vi "ELVIS III v1.0 Configure AI Mode.vi"(8 "error in (no error)":errorcluster, 10 "AI Channel List":T1, 11 "myRIO FPGA Ref Out":T3) -> (0 "error out":errorcluster)   [LabVIEW 2021]
uses:
  <vilib>/myRIO/Common/Instrument Driver Framework/Utilities/typedefs/Generic FPGA Reference.ctl
  <vilib>/myRIO/Common/Instrument Driver Framework/myRIO v1.0/AI/typedefs/AI Channels List.ctl
  <vilib>/myRIO/Common/Instrument Driver Framework/myRIO v1.0/AI/typedefs/AI Channels Enum.ctl
  <vilib>/myRIO/Common/Instrument Driver Framework/ELVIS III v1.0/AI/typedefs/ELVIS III AI Channels FPGA Reference.ctl
  <vilib>/myRIO/Common/Instrument Driver Framework/ELVIS III v1.0/AI/vis/ELVIS III v1.0 AI Global.vi
  <vilib>/Utility/error.llb/Error Cluster From Error Code.vi
  <vilib>/rvi/errors/niLvFpgaAdjustHostInterfaceError.vi
  <vilib>/rvi/interface/nirviReadWriteControl/nirviReadWriteControl.xnode
  NiFpgaLv.dll
  <vilib>/rvi/interface/Simulation/niFpgaSimulationCallBeginRW.vi
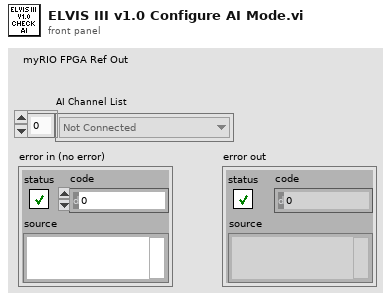
[diagram p1: front panel]
types:
  T1 = typedef "AI Channels List.ctl" = T2[]
  T2 = typedef "AI Channels Enum.ctl" = enum16{"Not Connected", "AudioIn/Left", "AudioIn/Right", "C/AI0", "C/AI1", "A/AI0", "A/AI1", "A/AI2", "A/AI3", "A/AI4", "A/AI5", "A/AI6", "A/AI7", "B/AI0", "B/AI1", "B/AI2", "B/AI3", "B/AI4", "B/AI5", "B/AI6", "B/AI7", "AI/AI0", "AI/AI1", "AI/AI2", "AI/AI3", "A/AI0 (DIFF)", "A/AI1 (DIFF)", "A/AI2 (DIFF)", "A/AI3 (DIFF)", "B/AI0 (DIFF)", "B/AI1 (DIFF)", "B/AI2 (DIFF)", "B/AI3 (DIFF)"}
  T3 = typedef "Generic FPGA Reference.ctl" = refnum<k20>
  T4 = typedef "ELVIS III AI Channels FPGA Reference.ctl" = refnum<k20>
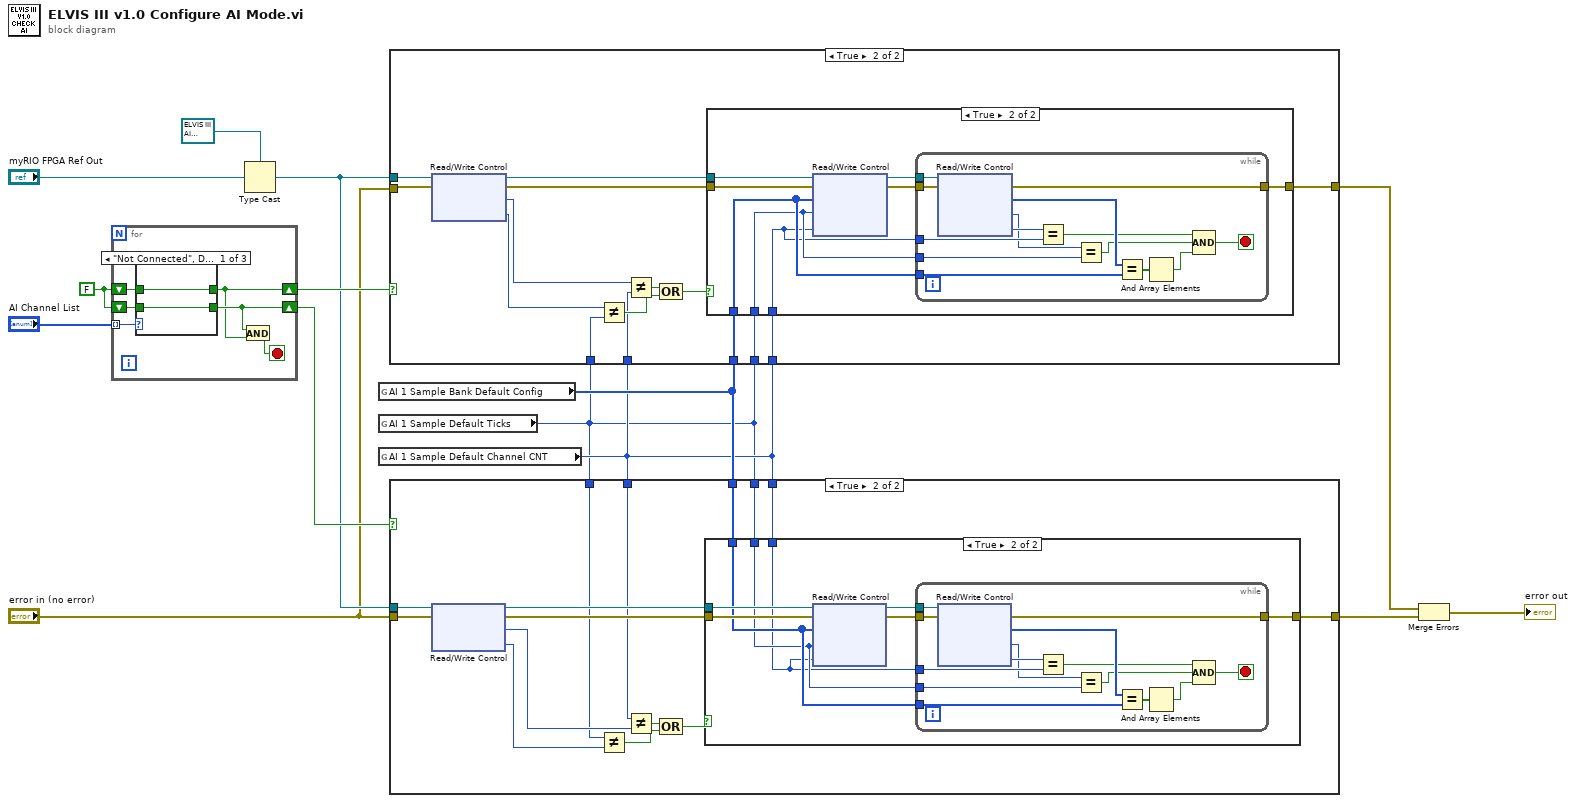
[diagram p0: block diagram]
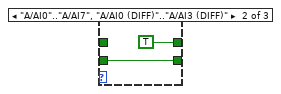
[diagram p6: hidden frame]
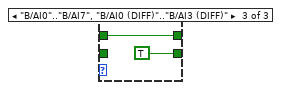
[diagram p7: hidden frame]
diagram:
  w11 = FALSE
  n1 = for {
    tunnel: "AI Channel List" -> [w20] mode=indexing
    shift-right: [w16] -> w10
    shift-left: w11 -> [w18]
    shift-right: [w17] -> w9
    shift-left: w11 -> [w19]
    stop <- w15 stop-if-true
    n2 = case shown="\"Not Connected\", Default" w20 {
      tunnel: w19 -> [w21 w24 _]
      tunnel: [w21 w24 TRUE] -> w17
      tunnel: w18 -> [w22 _ w25]
      tunnel: [w22 TRUE w25] -> w16
      frame "Not Connected", Default {
      }
      frame "A/AI0".."A/AI7", "A/AI0 (DIFF)".."A/AI3 (DIFF)" {
      }
      frame "B/AI0".."B/AI7", "B/AI0 (DIFF)".."B/AI3 (DIFF)" {
      }
    }
    n3 = And(x=w17, y=w16) -> (x .and. y?=w15:bool)
  }
  n4 = Type Cast(type=T4 refnum ("ELVIS III AI Channels FPGA Interface"), x="myRIO FPGA Ref Out") -> (*(type *) &x=w8:T4)
  n5 = global read "ELVIS III v1.0 AI Global.vi" "AI 1 Sample Bank Default Config"() -> (w3:u8[])
  n6 = global read "ELVIS III v1.0 AI Global.vi" "AI 1 Sample Default Ticks"() -> (w1:u32)
  n7 = global read "ELVIS III v1.0 AI Global.vi" "AI 1 Sample Default Channel CNT"() -> (w2:u8)
  n8 = case shown="True" w10 {
    tunnel: "error in (no error)" -> [w27 w41]
    tunnel: [w27 w33] -> w6
    tunnel: w8 -> [_ w40]
    tunnel: w3 -> [_ w32]
    tunnel: w1 -> [_ w31]
    tunnel: w2 -> [_ w30]
    tunnel: w2 -> [_ w29]
    tunnel: w1 -> [_ w28]
    frame False {
    }
    frame True {
      n9 = xnode "Read/Write Control"("FPGA VI Reference In"=w40, "error in"=w41) -> ("FPGA VI Reference Out"=w35:T4, "error out"=w34:errorcluster, "AI.A.CNT"=w42:u8, "AI.A.CNTR"=w39:u32)
      n10 = Not Equal?(x=w39, y=w28) -> (x != y?=w37:bool)
      n11 = Not Equal?(x=w42, y=w29) -> (x != y?=w38:bool)
      n12 = Compound Arithmetic op=OR(w38, w37) -> (w36:bool)
      n13 = case shown="True" w36 {
        tunnel: w35 -> [_ w51]
        tunnel: w34 -> [w43 w50]
        tunnel: [w43 w47] -> w33
        tunnel: w32 -> [_ w46]
        tunnel: w31 -> [_ w45]
        tunnel: w30 -> [_ w44]
        frame False {
        }
        frame True {
          n14 = xnode "Read/Write Control"("FPGA VI Reference In"=w51, "error in"=w50, "AI.A.CNFG"=w46, "AI.A.CNTR"=w45, "AI.A.CNT"=w44) -> ("FPGA VI Reference Out"=w49:T4, "error out"=w48:errorcluster)
          n15 = while {
            tunnel: w49 -> [w65]
            tunnel: w48 -> [w64]
            tunnel: w44 -> [w62]
            tunnel: w46 -> [w60]
            tunnel: [w58] -> w47
            tunnel: w45 -> [w56]
            stop <- w52 stop-if-true
            n16 = xnode "Read/Write Control"("FPGA VI Reference In"=w65, "error in"=w64) -> ("error out"=w58:errorcluster, "AI.A.CNFG"=w61:u8[], "AI.A.CNTR"=w57:u32, "AI.A.CNT"=w63:u8)  [unwired: 1 out]
            n17 = Equal?(x=w63, y=w62) -> (x = y?=w55:bool)
            n18 = Equal?(x=w57, y=w56) -> (x = y?=w54:bool)
            n19 = Equal?(x=w61, y=w60) -> (x = y?=w59:bool[])
            n20 = And Array Elements(Boolean array=w59) -> (logical AND=w53:bool)
            n21 = Compound Arithmetic op=AND(w55, w54, w53) -> (w52:bool)
          }
        }
      }
    }
  }
  n22 = case shown="True" w9 {
    tunnel: [w66 w78] -> w5
    tunnel: w8 -> [_ w77]
    tunnel: "error in (no error)" -> [w66 w76]
    tunnel: w3 -> [_ w71]
    tunnel: w1 -> [_ w70]
    tunnel: w2 -> [_ w69]
    tunnel: w2 -> [_ w68]
    tunnel: w1 -> [_ w67]
    frame False {
    }
    frame True {
      n23 = xnode "Read/Write Control"("FPGA VI Reference In"=w77, "error in"=w76) -> ("FPGA VI Reference Out"=w80:T4, "error out"=w79:errorcluster, "AI.B.CNT"=w81:u8, "AI.B.CNTR"=w75:u32)
      n24 = Not Equal?(x=w67, y=w75) -> (x != y?=w73:bool)
      n25 = Not Equal?(x=w68, y=w81) -> (x != y?=w74:bool)
      n26 = Compound Arithmetic op=OR(w74, w73) -> (w72:bool)
      n27 = case shown="True" w72 {
        tunnel: w80 -> [_ w90]
        tunnel: w79 -> [w82 w89]
        tunnel: [w82 w86] -> w78
        tunnel: w71 -> [_ w85]
        tunnel: w70 -> [_ w84]
        tunnel: w69 -> [_ w83]
        frame False {
        }
        frame True {
          n28 = xnode "Read/Write Control"("FPGA VI Reference In"=w90, "error in"=w89, "AI.B.CNFG"=w85, "AI.B.CNTR"=w84, "AI.B.CNT"=w83) -> ("FPGA VI Reference Out"=w88:T4, "error out"=w87:errorcluster)
          n29 = while {
            tunnel: w88 -> [w104]
            tunnel: w87 -> [w103]
            tunnel: w83 -> [w101]
            tunnel: w85 -> [w99]
            tunnel: [w97] -> w86
            tunnel: w84 -> [w95]
            stop <- w91 stop-if-true
            n30 = xnode "Read/Write Control"("FPGA VI Reference In"=w104, "error in"=w103) -> ("error out"=w97:errorcluster, "AI.B.CNFG"=w100:u8[], "AI.B.CNTR"=w96:u32, "AI.B.CNT"=w102:u8)  [unwired: 1 out]
            n31 = Equal?(x=w102, y=w101) -> (x = y?=w94:bool)
            n32 = Equal?(x=w96, y=w95) -> (x = y?=w93:bool)
            n33 = Equal?(x=w100, y=w99) -> (x = y?=w98:bool[])
            n34 = And Array Elements(Boolean array=w98) -> (logical AND=w92:bool)
            n35 = Compound Arithmetic op=AND(w94, w93, w92) -> (w91:bool)
          }
        }
      }
    }
  }
  n36 = Merge Errors(w6, w5) -> (→"error out":errorcluster)
